vi "Info schreiben.vi"(0 "Spaninlet":i32, 7 "Spangaseinstellungen":T2[](array[typedef]) {"Komponenten"."Komponente 5"."Komponente:" items=["NO (350,3000) LP 191C", "NO2 (150) LP 191C (1of2)", "NO2 (2000) LP 191C (2of2)", "N2O (300) LP 191C (1of2)", "NH3 (300) LP 191C (1of2)", "NH3 (900,3000) LP 191C (2of2)", "HNCO (400) 191C", "H2O% (30) LP 191C", "Formaldehyde (70,500) LP 191C", "CO2 low% (4) LP 191C (2of2)", "CO2% (20) LP 191C (1of2)", "CO (700) LP 191C (1of3)", "CO% (1) LP 191C (2of3)", "Propylene (1000) LP 191C", "Aromatic HC C7 (500) LP 191C", "Ethylene (1000) LP 191C", "CH4 (250) LP 191C (1of2)", "CH4 (5000) LP 191C (2of2)", "Ethane (1000) LP 191C", "Acetylene (1000) LP 191C", "HNO2 (20) 191C", "MeOH (1000) 191C", "CO% (10) LP 191C (3of3)", "Formic Acid (100) 191C", "SO2 (500) LP 191C", "Acetaldehyde (1000) LP 191C", "COS (100) LP 191C", "1,3 butadiene (100) LP 191C", "Oil as Octane (200) LP 191C", "N2O (1000) LP 191C (2of2)", "Propane (200) LP 191C", "NO2 autorange (2000)", "CO autorange (100000)", "CH4 autorange (5000)", "NH3 autorange (3000)", "Temp. Gascell", "Pressure Gascell", "sBeam@2500"]; "Komponenten"."Komponente 5"."Konzentration IST" format="%#.4f"; "Komponenten"."Komponente 5"."Genauigkeit" format="%#.1f"; "Komponenten"."Komponente 4"."Komponente:" items=["NO (350,3000) LP 191C", "NO2 (150) LP 191C (1of2)", "NO2 (2000) LP 191C (2of2)", "N2O (300) LP 191C (1of2)", "NH3 (300) LP 191C (1of2)", "NH3 (900,3000) LP 191C (2of2)", "HNCO (400) 191C", "H2O% (30) LP 191C", "Formaldehyde (70,500) LP 191C", "CO2 low% (4) LP 191C (2of2)", "CO2% (20) LP 191C (1of2)", "CO (700) LP 191C (1of3)", "CO% (1) LP 191C (2of3)", "Propylene (1000) LP 191C", "Aromatic HC C7 (500) LP 191C", "Ethylene (1000) LP 191C", "CH4 (250) LP 191C (1of2)", "CH4 (5000) LP 191C (2of2)", "Ethane (1000) LP 191C", "Acetylene (1000) LP 191C", "HNO2 (20) 191C", "MeOH (1000) 191C", "CO% (10) LP 191C (3of3)", "Formic Acid (100) 191C", "SO2 (500) LP 191C", "Acetaldehyde (1000) LP 191C", "COS (100) LP 191C", "1,3 butadiene (100) LP 191C", "Oil as Octane (200) LP 191C", "N2O (1000) LP 191C (2of2)", "Propane (200) LP 191C", "NO2 autorange (2000)", "CO autorange (100000)", "CH4 autorange (5000)", "NH3 autorange (3000)", "Temp. Gascell", "Pressure Gascell", "sBeam@2500"]; "Komponenten"."Komponente 4"."Konzentration IST" format="%#.4f"; "Komponenten"."Komponente 4"."Genauigkeit" format="%#.1f"; "Komponenten"."Komponente 3"."Komponente:" items=["NO (350,3000) LP 191C", "NO2 (150) LP 191C (1of2)", "NO2 (2000) LP 191C (2of2)", "N2O (300) LP 191C (1of2)", "NH3 (300) LP 191C (1of2)", "NH3 (900,3000) LP 191C (2of2)", "HNCO (400) 191C", "H2O% (30) LP 191C", "Formaldehyde (70,500) LP 191C", "CO2 low% (4) LP 191C (2of2)", "CO2% (20) LP 191C (1of2)", "CO (700) LP 191C (1of3)", "CO% (1) LP 191C (2of3)", "Propylene (1000) LP 191C", "Aromatic HC C7 (500) LP 191C", "Ethylene (1000) LP 191C", "CH4 (250) LP 191C (1of2)", "CH4 (5000) LP 191C (2of2)", "Ethane (1000) LP 191C", "Acetylene (1000) LP 191C", "HNO2 (20) 191C", "MeOH (1000) 191C", "CO% (10) LP 191C (3of3)", "Formic Acid (100) 191C", "SO2 (500) LP 191C", "Acetaldehyde (1000) LP 191C", "COS (100) LP 191C", "1,3 butadiene (100) LP 191C", "Oil as Octane (200) LP 191C", "N2O (1000) LP 191C (2of2)", "Propane (200) LP 191C", "NO2 autorange (2000)", "CO autorange (100000)", "CH4 autorange (5000)", "NH3 autorange (3000)", "Temp. Gascell", "Pressure Gascell", "sBeam@2500"]; "Komponenten"."Komponente 3"."Konzentration IST" format="%#.4f"; "Komponenten"."Komponente 3"."Genauigkeit" format="%#.1f"; "Komponenten"."Komponente 2"."Komponente:" items=["NO (350,3000) LP 191C", "NO2 (150) LP 191C (1of2)", "NO2 (2000) LP 191C (2of2)", "N2O (300) LP 191C (1of2)", "NH3 (300) LP 191C (1of2)", "NH3 (900,3000) LP 191C (2of2)", "HNCO (400) 191C", "H2O% (30) LP 191C", "Formaldehyde (70,500) LP 191C", "CO2 low% (4) LP 191C (2of2)", "CO2% (20) LP 191C (1of2)", "CO (700) LP 191C (1of3)", "CO% (1) LP 191C (2of3)", "Propylene (1000) LP 191C", "Aromatic HC C7 (500) LP 191C", "Ethylene (1000) LP 191C", "CH4 (250) LP 191C (1of2)", "CH4 (5000) LP 191C (2of2)", "Ethane (1000) LP 191C", "Acetylene (1000) LP 191C", "HNO2 (20) 191C", "MeOH (1000) 191C", "CO% (10) LP 191C (3of3)", "Formic Acid (100) 191C", "SO2 (500) LP 191C", "Acetaldehyde (1000) LP 191C", "COS (100) LP 191C", "1,3 butadiene (100) LP 191C", "Oil as Octane (200) LP 191C", "N2O (1000) LP 191C (2of2)", "Propane (200) LP 191C", "NO2 autorange (2000)", "CO autorange (100000)", "CH4 autorange (5000)", "NH3 autorange (3000)", "Temp. Gascell", "Pressure Gascell", "sBeam@2500"]; "Komponenten"."Komponente 2"."Konzentration IST" format="%#.4f"; "Komponenten"."Komponente 2"."Genauigkeit" format="%#.1f"; "Komponenten"."Komponente 1"."Komponente:" items=["NO (350,3000) LP 191C", "NO2 (150) LP 191C (1of2)", "NO2 (2000) LP 191C (2of2)", "N2O (300) LP 191C (1of2)", "NH3 (300) LP 191C (1of2)", "NH3 (900,3000) LP 191C (2of2)", "HNCO (400) 191C", "H2O% (30) LP 191C", "Formaldehyde (70,500) LP 191C", "CO2 low% (4) LP 191C (2of2)", "CO2% (20) LP 191C (1of2)", "CO (700) LP 191C (1of3)", "CO% (1) LP 191C (2of3)", "Propylene (1000) LP 191C", "Aromatic HC C7 (500) LP 191C", "Ethylene (1000) LP 191C", "CH4 (250) LP 191C (1of2)", "CH4 (5000) LP 191C (2of2)", "Ethane (1000) LP 191C", "Acetylene (1000) LP 191C", "HNO2 (20) 191C", "MeOH (1000) 191C", "CO% (10) LP 191C (3of3)", "Formic Acid (100) 191C", "SO2 (500) LP 191C", "Acetaldehyde (1000) LP 191C", "COS (100) LP 191C", "1,3 butadiene (100) LP 191C", "Oil as Octane (200) LP 191C", "N2O (1000) LP 191C (2of2)", "Propane (200) LP 191C", "NO2 autorange (2000)", "CO autorange (100000)", "CH4 autorange (5000)", "NH3 autorange (3000)", "Temp. Gascell", "Pressure Gascell", "sBeam@2500"]; "Komponenten"."Komponente 1"."Konzentration IST" format="%#.4f"; "Komponenten"."Komponente 1"."Genauigkeit" format="%#.1f"; "Modus" items=["Cal Gas to PNS", "Cal Gas to Samplepoint"]; "Ablaufdatum" format="%<%d.%m.%Y>T"; "Gasflasche" items=["----"=10000, "IAG NH3 3000"=0, "IAG NH3 200"=1, "IAG NH3 2000"=2, "IAG MG"=3, "IAG O2"=4]}, 11 "error in (no error)":errorcluster caption="Fehler (Eingang, kein Fehler)") -> (4 "Array":T1[][](array[typedef]), 15 "error out":errorcluster caption="Fehler (Ausgang)")   [LabVIEW 2020, in "EPA 1065.lvlib" / "Gas Analyzer Drift 1065-550.lvlib"]
uses:
  Gas Analyzer Drift 1065-550.lvlib
  Spaninlet Cluster.ctl
  Seiten/System Einstellungen V2/Konfig Gasflasche.ctl
  Seiten/System Einstellungen V2/Analysatoren.ctl
  Seiten/System Einstellungen V2/Gasflasche Auswahl.ctl
  T90 1065-308/Modus.ctl
  Komponentencluster.ctl
  Komponentenauswahl.ctl
  Visualisierungs Elemente/String - Ausgabefeld.ctl
  Seiten/FT-IR/FGV FT-IR Gasliste Aktionen.ctl
  Seiten/FT-IR/FT-IR.lvlib
  Seiten/System Einstellungen V2/System Einstellungen V2.lvlib
  T90 1065-308/T90 Test 1065-308.lvlib
panel:
  # "Komponente"
  # "Konzentration"
  # "Einheit"
  # "Genauigkeit [%]"
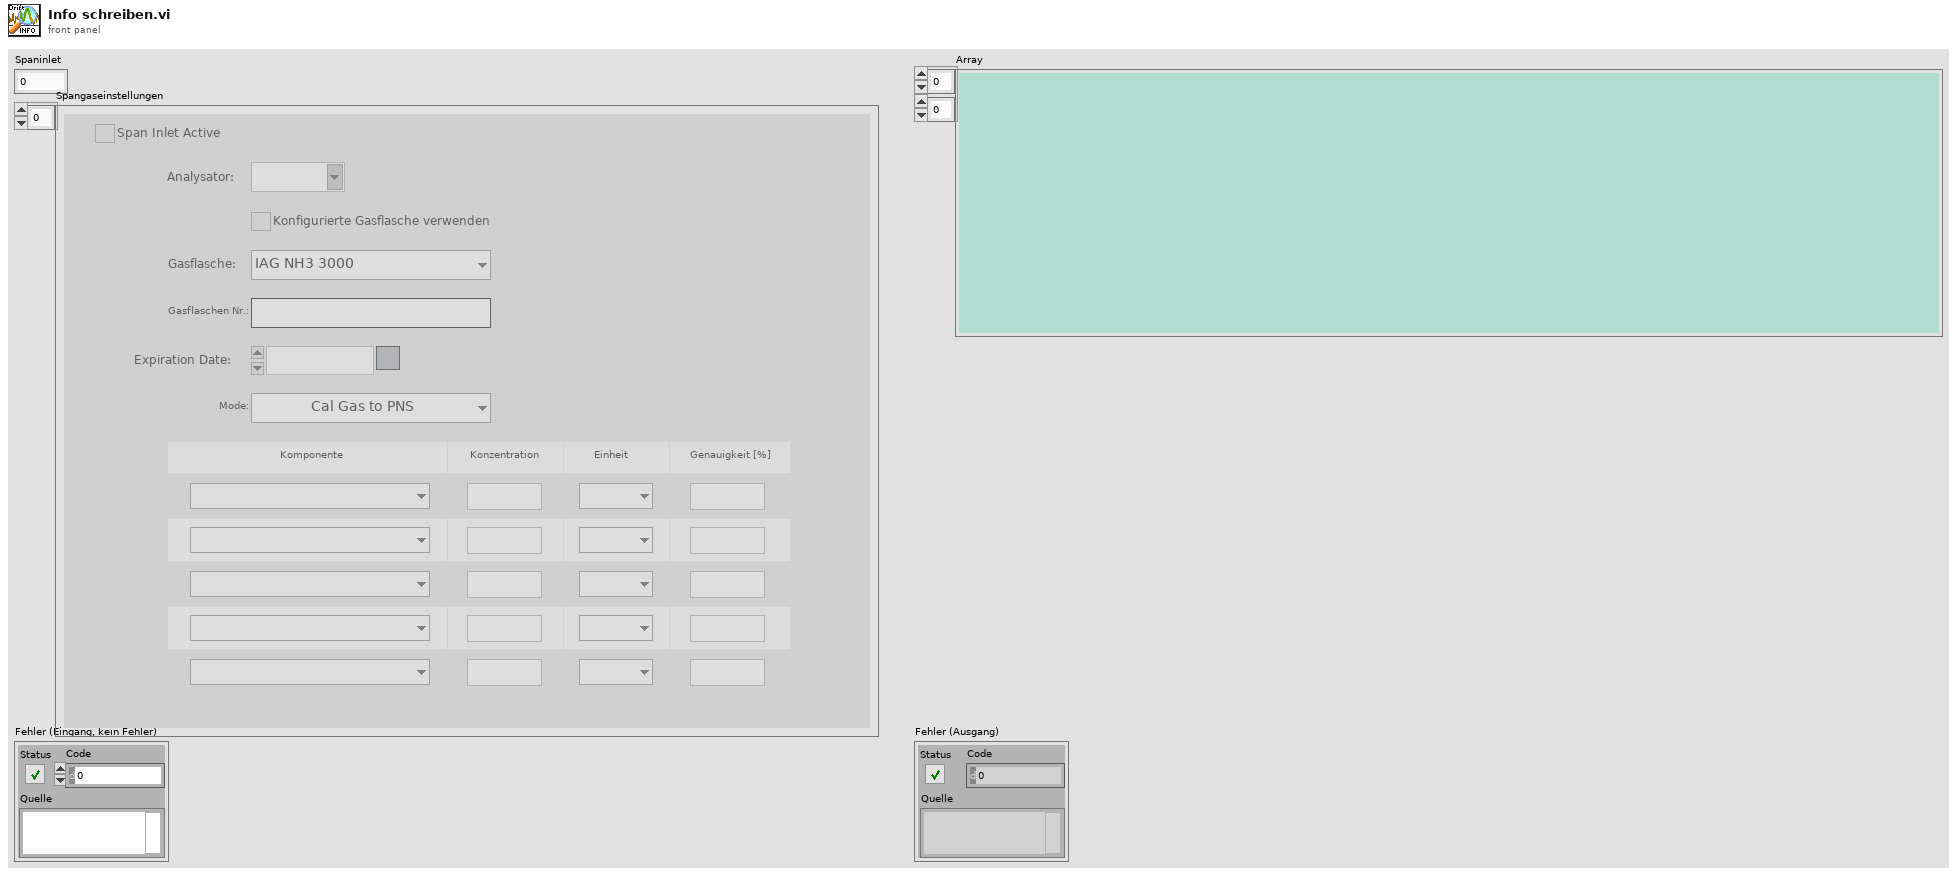
[diagram p1: front panel]
types:
  T1 = typedef "String - Ausgabefeld.ctl" = string
  T2 = typedef "EPA 1065.lvlib/Gas Analyzer Drift 1065-550.lvlib/Spaninlet Cluster.ctl" = cluster{"Span Inlet Active":T3, "Analysator":T4, "Konfig Gasflasche":T3, "Gasflasche":T5, "Gasflaschen Nr.:":string, "Ablaufdatum":timestamp, "Modus":T6, "Komponenten":T7}
  T3 = typedef "System Einstellungen V2.lvlib/Konfig Gasflasche.ctl" = bool
  T4 = typedef "System Einstellungen V2.lvlib/Analysatoren.ctl" = string
  T5 = typedef "System Einstellungen V2.lvlib/Gasflasche Auswahl.ctl" = u16
  T6 = typedef "EPA 1065.lvlib/T90 Test 1065-308.lvlib/Modus.ctl" = u16
  T7 = typedef "EPA 1065.lvlib/Gas Analyzer Drift 1065-550.lvlib/Komponentencluster.ctl" = cluster{"Komponente 1":T8, "Komponente 2":T8, "Komponente 3":T8, "Komponente 4":T8, "Komponente 5":T8}
  T8 = typedef "EPA 1065.lvlib/Gas Analyzer Drift 1065-550.lvlib/Komponentenauswahl.ctl" = cluster{"Komponente:":u16, "Konzentration IST":dbl, "Einheit":enum16{"ppm", "%"}, "Genauigkeit":dbl}
  T9 = typedef "FT-IR.lvlib/FGV FT-IR Gasliste Aktionen.ctl" = enum16{"lesen", "Gasliste FT-IR", "Gasliste ausgelesen", "laden", "speichern", "löschen"}
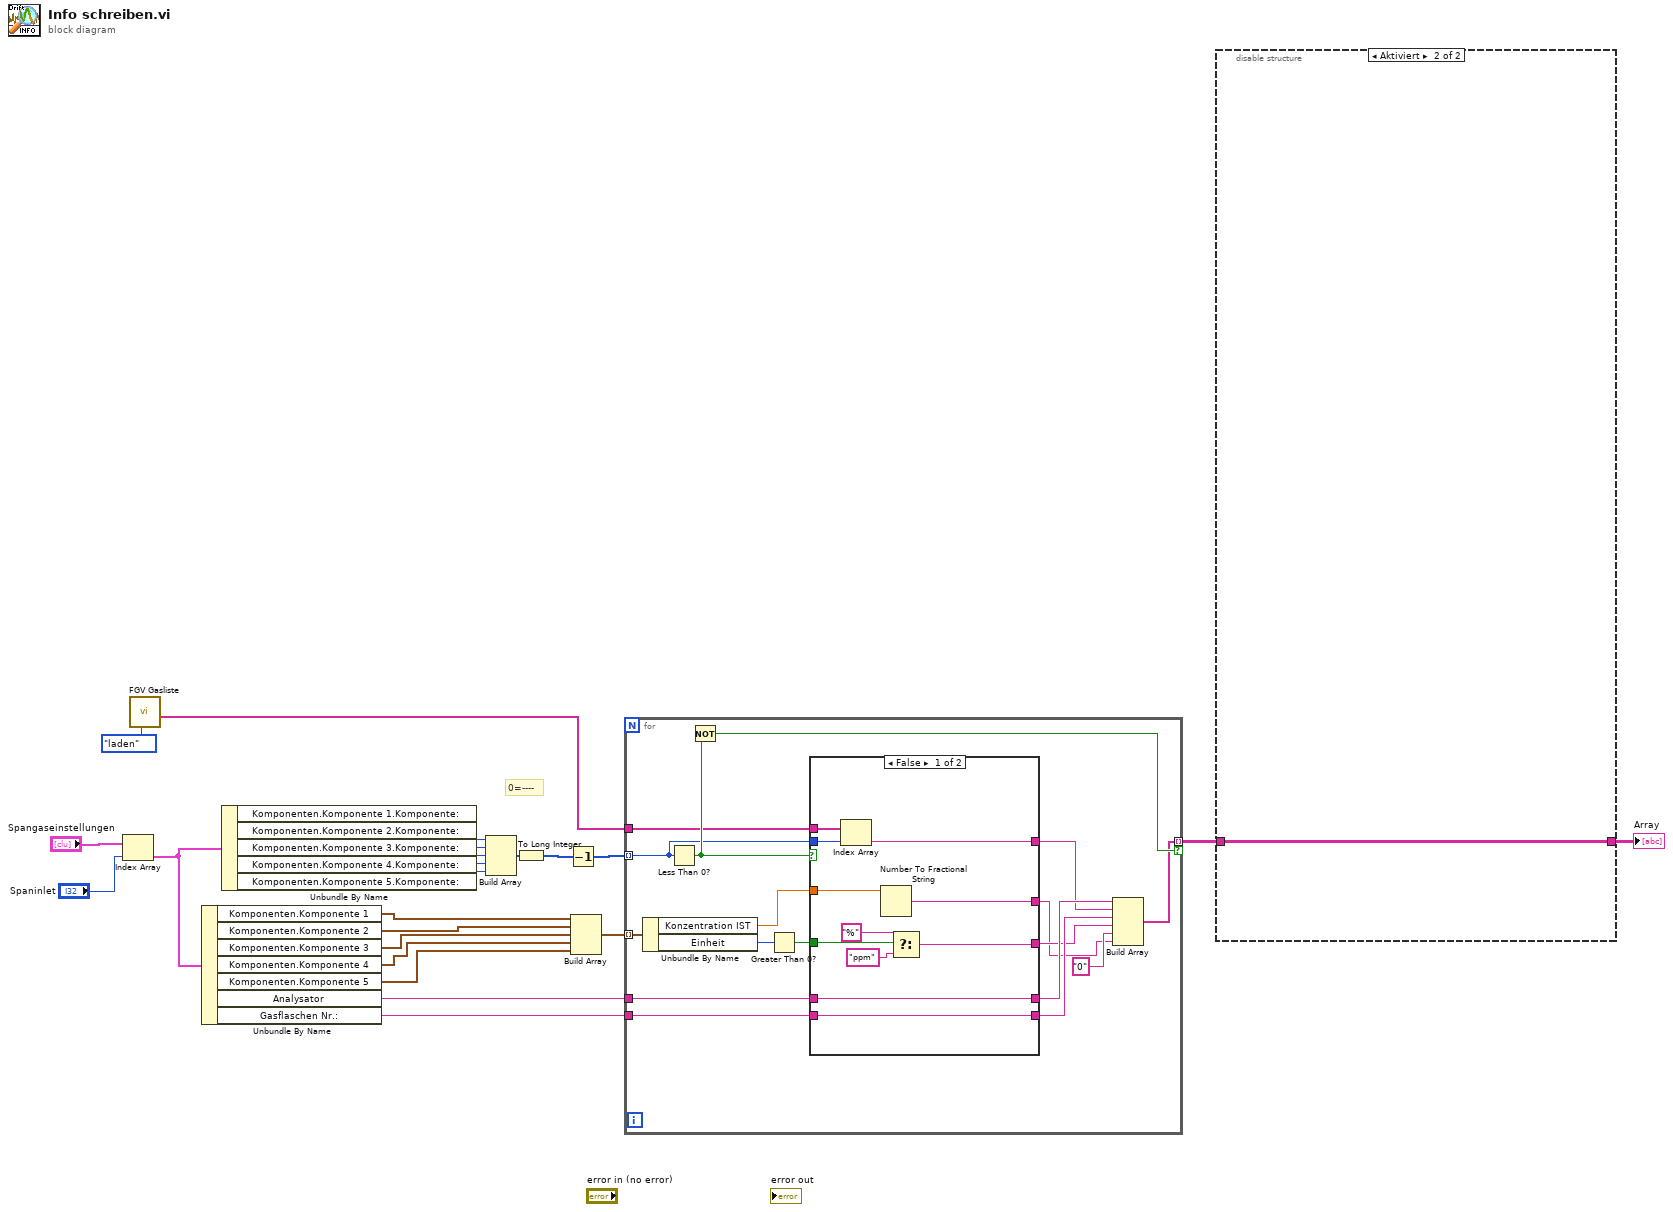
[diagram p0: block diagram]
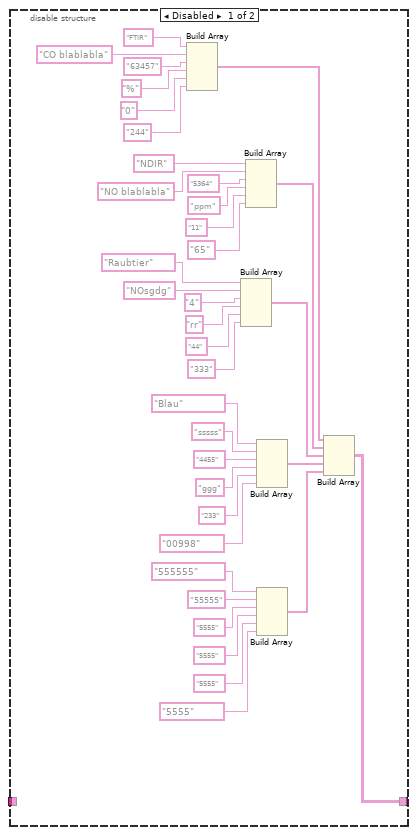
[diagram p2: hidden frame]
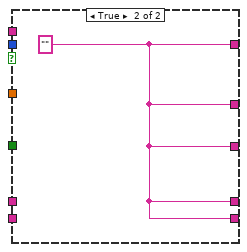
[diagram p3: hidden frame]
diagram:
  # "0=----"
  n1 = Index Array(array="Spangaseinstellungen", index="Spaninlet") -> (element=w7:T2)
  n2 = call "FGV Gasliste.vi"("Aktionen"=FGV_FT-IR_Gasliste_Aktionen."laden") -> ("Aktuelle Gasliste gesamt"=w13:T1[])  [unwired: 8 in, 2 out]
  n3 = Unbundle By Name(w7) -> ("Komponenten.Komponente 1"=w12:T8, "Komponenten.Komponente 2"=w11:T8, "Komponenten.Komponente 3"=w10:T8, "Komponenten.Komponente 4"=w9:T8, "Komponenten.Komponente 5"=w8:T8, "Analysator"=w5:T4, "Gasflaschen Nr.:"=w4:string)
  n4 = Unbundle By Name(w7) -> ("Komponenten.Komponente 1.Komponente:"=w21:u16, "Komponenten.Komponente 2.Komponente:"=w20:u16, "Komponenten.Komponente 3.Komponente:"=w19:u16, "Komponenten.Komponente 4.Komponente:"=w18:u16, "Komponenten.Komponente 5.Komponente:"=w17:u16)
  n5 = Build Array(w21, w20, w19, w18, w17) -> (w16:u16[])
  n6 = To Long Integer(number=w16) -> (32bit integer=w3:i32[])
  n7 = Decrement(x=w3) -> (x-1=w15:i32[])
  n8 = Build Array(w12, w11, w10, w9, w8) -> (w6:T8[])
  n9 = for {
    tunnel: [w24] -> w2 mode=indexing if=w39
    tunnel: w15 -> [w38] mode=indexing
    tunnel: w13 -> [w37]
    tunnel: w6 -> [w36] mode=indexing
    tunnel: w5 -> [w32]
    tunnel: w4 -> [w31]
    n10 = Unbundle By Name(w36) -> ("Konzentration IST"=w35:dbl, "Einheit"=w33:enum16{"ppm", "%"})
    n11 = Less Than 0?(x=w38) -> (x < 0?=w40:bool)
    n12 = Not(x=w40) -> (.not. x?=w39:bool)
    n13 = Greater Than 0?(x=w33) -> (x > 0?=w34:bool)
    n14 = case shown="False" w40 {
      tunnel: [w49 w52] -> w29
      tunnel: w38 -> [w50 _]
      tunnel: w37 -> [w51 _]
      tunnel: w35 -> [w48 _]
      tunnel: w34 -> [w45 _]
      tunnel: w32 -> [w44 _]
      tunnel: w31 -> [w43 _]
      tunnel: [w44 w52] -> w30
      tunnel: [w43 w52] -> w28
      tunnel: [w42 w52] -> w27
      tunnel: [w41 w52] -> w25
      frame False {
        n15 = Index Array(array=w51, index=w50) -> (element=w49:T1)
        n16 = Number To Fractional String(number=w48) -> (F-format string=w41:string)  [unwired: 3 in]
        n17 = Select(t="%", s=w45, f="ppm") -> (s? t:f=w42:string)
      }
      frame True {
        w52 = T1 "" ("String - Ausgabefeld")
      }
    }
    n18 = Build Array(w30, w29, w28, w27, T1 "0" ("Element"), w25) -> (w24:T1[])
  }
  n19 = disable-structure shown="Aktiviert" {
    disable-tunnel: w2 -> [_ w89]
    disable-tunnel: [w53 w89] -> w1
    frame Disabled {
      n20 = Build Array(T1 "FTIR" ("String - Ausgabefeld"), T1 "CO blablabla" ("String - Ausgabefeld"), T1 "63457" ("String - Ausgabefeld"), T1 "%" ("String - Ausgabefeld"), T1 "0" ("Element"), T1 "244" ("Element")) -> (w58:T1[])
      n21 = Build Array(T1 "Raubtier" ("String - Ausgabefeld"), T1 "NOsgdg" ("String - Ausgabefeld"), T1 "4" ("String - Ausgabefeld"), T1 "rr" ("String - Ausgabefeld"), T1 "44" ("Element"), T1 "333" ("Element")) -> (w56:T1[])
      n22 = Build Array(T1 "NDIR" ("String - Ausgabefeld"), T1 "NO blablabla" ("String - Ausgabefeld"), T1 "5364" ("String - Ausgabefeld"), T1 "ppm" ("String - Ausgabefeld"), T1 "11" ("Element"), T1 "65" ("Element")) -> (w57:T1[])
      n23 = Build Array(T1 "Blau" ("String - Ausgabefeld"), T1 "sssss" ("String - Ausgabefeld"), T1 "4455" ("String - Ausgabefeld"), T1 "ggg" ("String - Ausgabefeld"), T1 "233" ("Element"), T1 "00998" ("Element")) -> (w55:T1[])
      n24 = Build Array(T1 "555555" ("String - Ausgabefeld"), T1 "55555" ("String - Ausgabefeld"), T1 "5555" ("String - Ausgabefeld"), T1 "5555" ("String - Ausgabefeld"), T1 "5555" ("Element"), T1 "5555" ("Element")) -> (w54:T1[])
      n25 = Build Array(w58, w57, w56, w55, w54) -> (w53:T1[][])
    }
    frame Enabled {
    }
  }
  "Array" <- w1
